vi "subtransform.vi"(5 "PairedCoordinatesShifted":T2[](array[typedef]), 6 "PairedFiducialCoordinates":T2[](array[typedef]), 7 "C":T1) -> (1 "size(s)":i32[](array[numeric]), 2 "A":T1, 3 "error":i32 format="%.3p", 4 "B":T1)   [LabVIEW 2011]
doc: "Calculate the coordinate transform given the Paired Fiducials.\n\nFirst using the shifted coordinates so they have a common point of rotation about the origin for the scaling a rotation matrix (namely the first paired fiducial in the list) form a 2D array of both reference and current session pair fiducials. The shift was performed by the calling routine. Both the shifted and orginal paired coordinates and C the shift vector are passed into this routine. All could have been done from the original paired fiducial coordinates structure.\n\nR = [ xr1, yr1, zr1\n xr2, yr2, zr2\n xr3, yr3, zr3\n .... ]\n\nY = [x1, y1 z1\n x2 y2 z2\n x3 y3 z3\n .... ]\n\nWhere Y are the shifted coordinates for the current session\nand R are the shifted coordinates for the reference session.\n\nFind A: Since Y = A* R then A = Y*inv(R) where inv is a psuedo inverse if the system of equations is overdetermined forming a least squares solution to the inverse.\n\nThen sove for B the shift of the out put as average offset of the shifted reference fidicuials transformed by the calculated A and the current session locations unsifted."
uses:
  <vilib>/Analysis/Matrix/Datatypes/RealMatrix.ctl
  Fiducial_pair.ctl
  <vilib>/Analysis/Matrix/NI_Matrix.lvlib
panel:
  # "Fiducial Location Pair"
  # "Current Instrument Fiducial Location"
  # "Reference Instrument Fiducial Location"
  # "Fiducial Location Pair"
  # "Current Instrument Fiducial Location"
  # "Reference Instrument Fiducial Location"
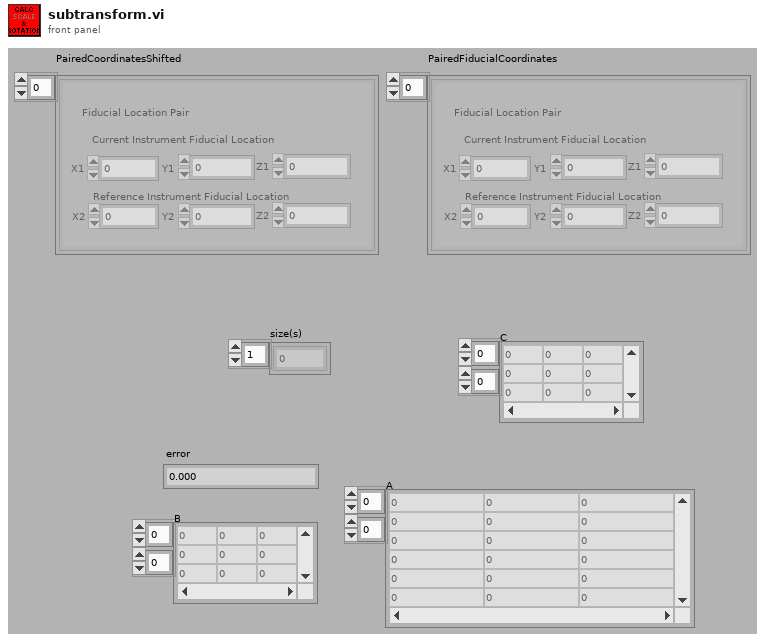
[diagram p1: front panel]
types:
  T1 = typedef "NI_Matrix.lvlib/RealMatrix.ctl" = dbl[][]
  T2 = typedef "Fiducial_pair.ctl" = cluster{"X1":dbl, "X2":dbl, "Y1":dbl, "Y2":dbl, "Z1":dbl, "Z2":dbl}
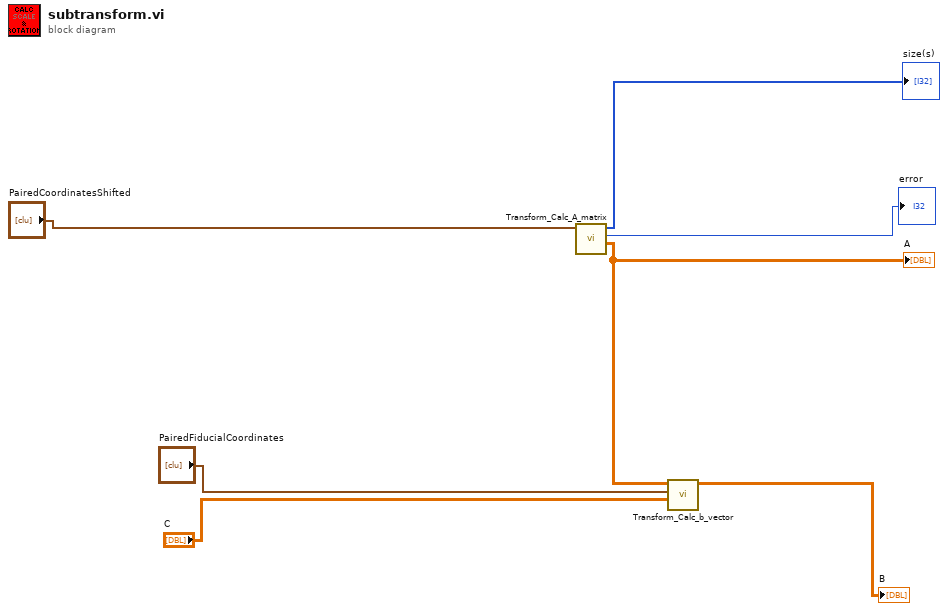
[diagram p0: block diagram]
diagram:
  n1 = call "Transform_Calc_A_matrix.vi"("PairedCoordinatesShifted"="PairedCoordinatesShifted") -> ("A"=w1:T1, "error"=→"error":i32, "Array"=→"size(s)":i32[])  [unwired: 8 in]
  "A" <- w1
  n2 = call "Transform_Calc_b_vector.vi"("C"="C", "PairedFiducialCoordinates"="PairedFiducialCoordinates", "A"=w1) -> ("b"=→"B":T1)  [unwired: 8 in]
